vi "Set Values.vi"(8 "error in":errorcluster, 10 "Values":refnum<class "Value.lvclass">[](array[class]), 11 "Object Entry in":refnum<class "Section.lvclass">) -> (0 "error out":errorcluster, 3 "Object Entry out":refnum<class "Section.lvclass">)   [LabVIEW 2024, in "Electronic Datasheet.lvlib" / "Section.lvclass"]
uses:
  Section.lvclass
  Value/Value.lvclass
  Section.lvclass/Section.ctl
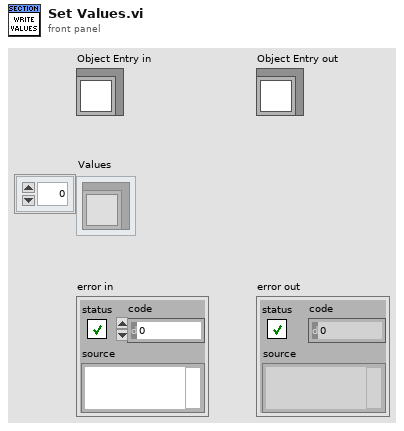
[diagram p1: front panel]
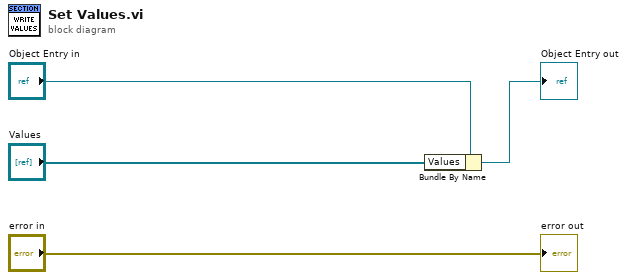
[diagram p0: block diagram]
diagram:
  n1 = Bundle By Name(cluster="Object Entry in", "Values"="Values") -> (→"Object Entry out":refnum<class "Section.lvclass">)
  "error out" <- "error in"
